vi "Write Integrate Configuration.vi"(8 "error in (no error)":errorcluster, 10 "Configuration":T1={"Integrate"=[], "Offset duration "=0.0095} {"Integrate"."Duration" format="%#_6p"; "Integrate"."Start time" format="%#_6p"}, 11 "Integrate in":refnum<class "Integrate.lvclass">) -> (0 "error out":errorcluster, 3 "Integrate out":refnum<class "Integrate.lvclass">)   [LabVIEW 2015, in "Integrate.lvclass"]
uses:
  Integrate.lvclass
  Integrator Configoration.ctl
  NHMFL_Core/Libraries/Utilities/Controls/Integrate channel.ctl
  Measure_core/Measure Object/Measure Object.lvclass/Measure Object.ctl
  Measure_core/Measure Object/Write Configuration.vi
panel:
  # "Input CH            Factor      Output CH      Start         Duration"
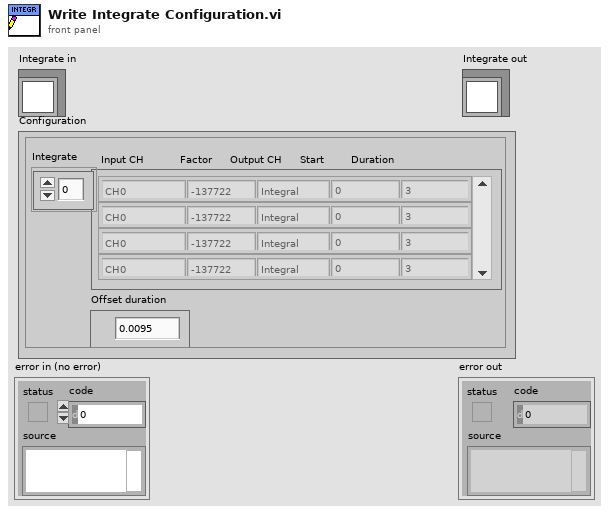
[diagram p1: front panel]
types:
  T1 = typedef "Integrator Configoration.ctl" = cluster{"Integrate":T2[], "Offset duration ":dbl}
  T2 = typedef "Integrate channel.ctl" = cluster{"Channel":string, "Output name":string, "Factor":dbl, "Start time":dbl, "Duration":dbl}
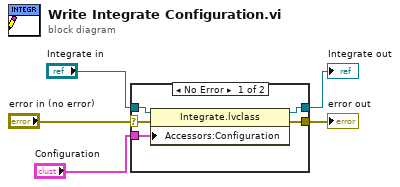
[diagram p0: block diagram]
diagram:
  n1 = case shown="No Error" "error in (no error)" {
    selector: "error in (no error)" -> [w7 w11]
    tunnel: [w6 w11] -> w4
    tunnel: [w9 w12] -> w2
    tunnel: "Integrate in" -> [w10 w12]
    tunnel: "Configuration" -> [w8 _]
    frame No Error {
      n2 = property class="Integrate.lvclass"(reference=w10, error in=w7, "Accessors:Configuration"=w8) -> (reference out=w9:refnum<class "Integrate.lvclass">, error out=w6:errorcluster)
    }
    frame Error {
    }
  }
  "error out" <- w4
  "Integrate out" <- w2
